vi "transform_inverse.vi"(1 "Transform":T1 format="%#.2f") -> (0 "Inverse transform":T1 format="%#.2f")   [LabVIEW 2013]
uses:
  <vilib>/Analysis/Matrix/Datatypes/RealMatrix.ctl
  <vilib>/Analysis/baseanly.llb/Real A x B.vi
  <vilib>/Analysis/NI_AALBase.lvlib
  <vilib>/Analysis/Matrix/NI_Matrix.lvlib
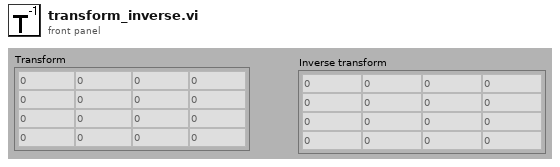
[diagram p1: front panel]
types:
  T1 = typedef "NI_Matrix.lvlib/RealMatrix.ctl" = dbl[][]
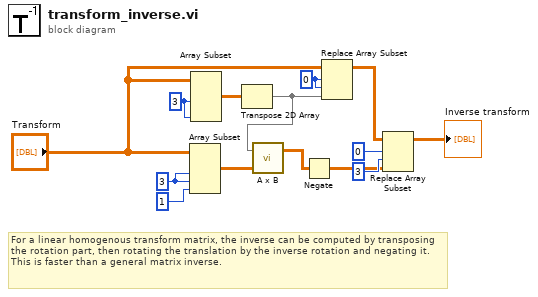
[diagram p0: block diagram]
diagram:
  w9 = 0 ("index (row)")
  w8 = 3 ("index")
  w5 = 3 ("length")
  # "For a linear homogenous transform matrix, the inverse can be computed by transposing the rotation part, then rotating the translation by the inverse rotation and negating it.  This is faster than a general matrix inverse."
  n1 = Array Subset(array="Transform", length (row)=w8, index (col)=w8, length (col)=1 ("length")) -> (w3:T1)  [unwired: 1 in]
  n2 = Array Subset(array="Transform", length (row)=w5, length (col)=w5) -> (w6:T1)  [unwired: 2 in]
  n3 = Transpose 2D Array(2D array=w6) -> (transposed array=w4:T1)
  n4 = call-poly <vilib>:"A x B.vi"("B"=w3, "A"=w4) -> ("A x B"=w1:T1)  [unwired: 1 out]
  n5 = Negate(x=w1) -> (-x=w10:T1)
  n6 = Replace Array Subset(array="Transform", new element=w4, index (row)=w9, index (col)=w9) -> (w11:T1)
  n7 = Replace Array Subset(array=w11, new element=w10, index (row)=0 ("disabled index (row)"), index (col)=3 ("disabled index (col)")) -> (→"Inverse transform":T1)
